vi "LvIRKit_SUB_Messages_POST.vi"(8 "error in (no error)":errorcluster, 10 "Message":string, 11 "IRKit IP address":string) -> (0 "error out":errorcluster)   [LabVIEW 2014]
uses:
  <vilib>/httpClient/POSTBuffer.vi
  <vilib>/httpClient/LabVIEWHTTPClient.lvlib
panel:
  # "LvIRKit:: Message POST"
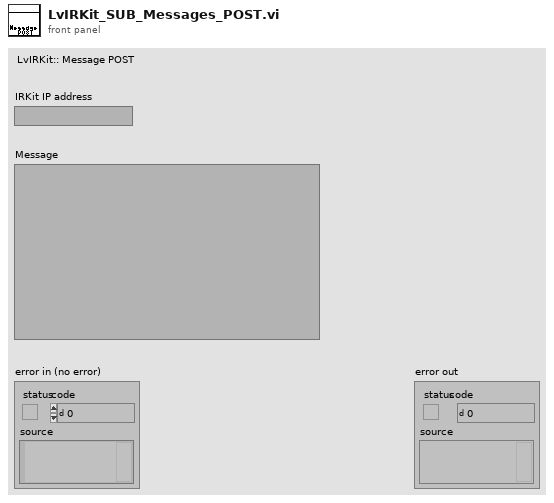
[diagram p1: front panel]
types:
  T1 = typedef "LabVIEWHTTPClient.lvlib/ClientHandle.ctl" = refnum<k1>
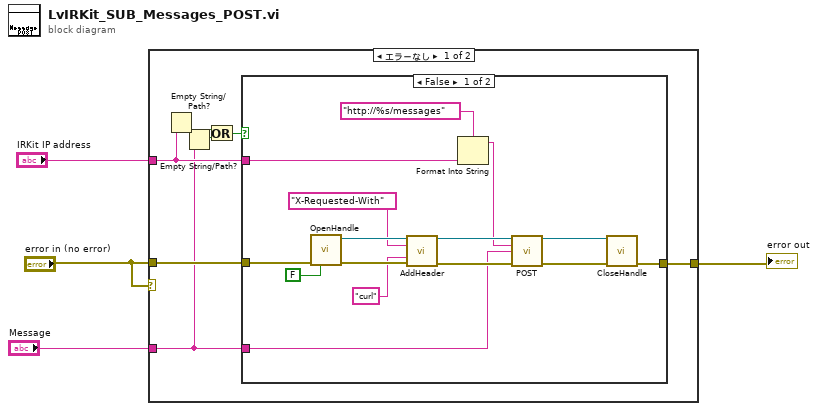
[diagram p0: block diagram]
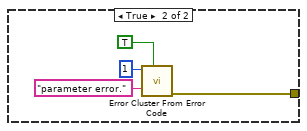
[diagram p2: hidden frame]
diagram:
  n1 = case shown="エラーなし" "error in (no error)" {
    tunnel: [w11 w31] -> w4
    tunnel: "error in (no error)" -> [w10 w31]
    tunnel: "Message" -> [w8 _]
    tunnel: "IRKit IP address" -> [w9 _]
    frame No Error {
      n2 = Empty String/Path?(string/path=w9) -> (empty?=w6:bool)
      n3 = Empty String/Path?(string/path=w8) -> (empty?=w7:bool)
      n4 = Or(x=w6, y=w7) -> (x .or. y?=w5:bool)
      n5 = case shown="FALSE" w5 {
        tunnel: [w15 w27] -> w11
        tunnel: w10 -> [w14 _]
        tunnel: w8 -> [w13 _]
        tunnel: w9 -> [w12 _]
        frame False {
          n6 = call <vilib>:"OpenHandle.vi"("error in (no error)"=w14, "verify server(true)"=FALSE) -> ("client handle out"=w23:T1, "error out"=w26:errorcluster)  [unwired: 12 in]
          n7 = call <vilib>:"AddHeader.vi"("client handle"=w23, "header"="X-Requested-With" ("url"), "value"="curl" ("url"), "error in (no error)"=w26) -> ("client handle out"=w24:T1, "error out"=w25:errorcluster)  [unwired: 10 in]
          n8 = Format Into String(format string="http://%s/messages", w12) -> (resulting string=w19:string)  [unwired: 2 in, 1 out]
          n9 = call-poly <vilib>:"POST.vi"("client handle"=w24, "url"=w19, "buffer"=w13, "error in (no error)"=w25) -> ("client handle out"=w17:T1, "error out"=w18:errorcluster)  [unwired: 8 in, 2 out]
          n10 = call <vilib>:"CloseHandle.vi"("client handle"=w17, "error in (no error)"=w18) -> ("error out"=w15:errorcluster)  [unwired: 13 in]
        }
        frame True {
          n11 = call <vilib>:"Error Cluster From Error Code.vi"("show call chain? (False)"=TRUE, "error message (\"\")"="parameter error." ("error message (\"\")"), "error code (0)"=1) -> ("error out"=w27:errorcluster)  [unwired: 6 in]
        }
      }
    }
    frame Error {
    }
  }
  "error out" <- w4
